vi "Initialise.vi"(8 "error in (no error)":errorcluster, 10 "Message in":refnum<class "InitialiseMessage.lvclass">, 11 "StageSPIM in":refnum<class "StageSPIM.lvclass">) -> (0 "error out":errorcluster, 3 "StageSPIM out":refnum<class "StageSPIM.lvclass">)   [LabVIEW 2012, in "StageSPIM.lvclass"]
doc: "This method is called when an initialise message is received. It mainly initialises the RabbitMQ connectivity. \n\nOverride this method when your component needs special initialisation (e.g. of software or hardware resources). In that case, don't forget to call the parent for proper implementation. If your component owns subcomponents, they count as resources, so you have to initialise them by calling their own initialise functions"
uses:
  StageSPIM.lvclass
  <vilib>/Distrio/Murmex/InitialiseMessage/InitialiseMessage.lvclass
  <vilib>/Distrio/Murmex/Murmex/Murmex.lvclass
  StageSPIM.lvclass/StageSPIM.ctl
panel:
  # "This method is called when the INTIALISE\ntrigger is sent. \n\nOverride this method when your component needs to\nrespond to this trigger. \n\nCall parent for proper implementation"
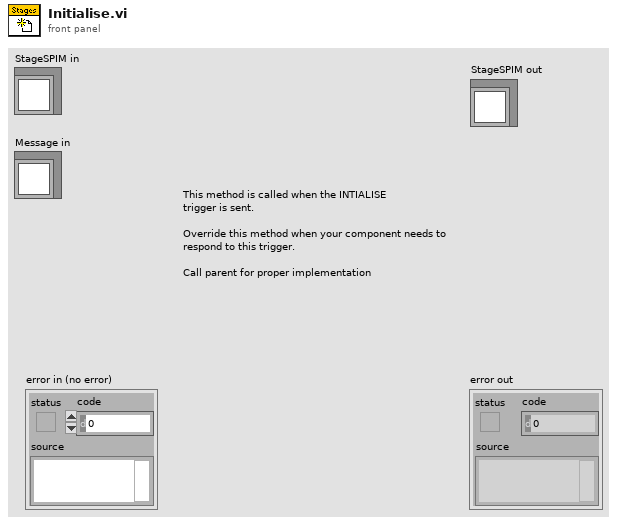
[diagram p1: front panel]
types:
  T1 = cluster{"Register DC":bool, "DaisyChain Search?":bool, "Device ID":i32}[][]
  T2 = cluster{"RON Affected axes":string[], "Reference mode":bool[], "Check FRF?":bool}
  T3 = typedef "StageSPIM.lvclass/port_control.ctl" = i32
  T4 = typedef "StageSPIM.lvclass/baud_rate_control.ctl" = u16
  T5 = typedef "StageSPIM.lvclass/connection_type.ctl" = enum16{"RS232", "RS232 DaisyChain", "USB", "USB_DaisyChain"}
  T6 = cluster{"Register DC":bool, "DaisyChain Search?":bool, "Device ID":i32}
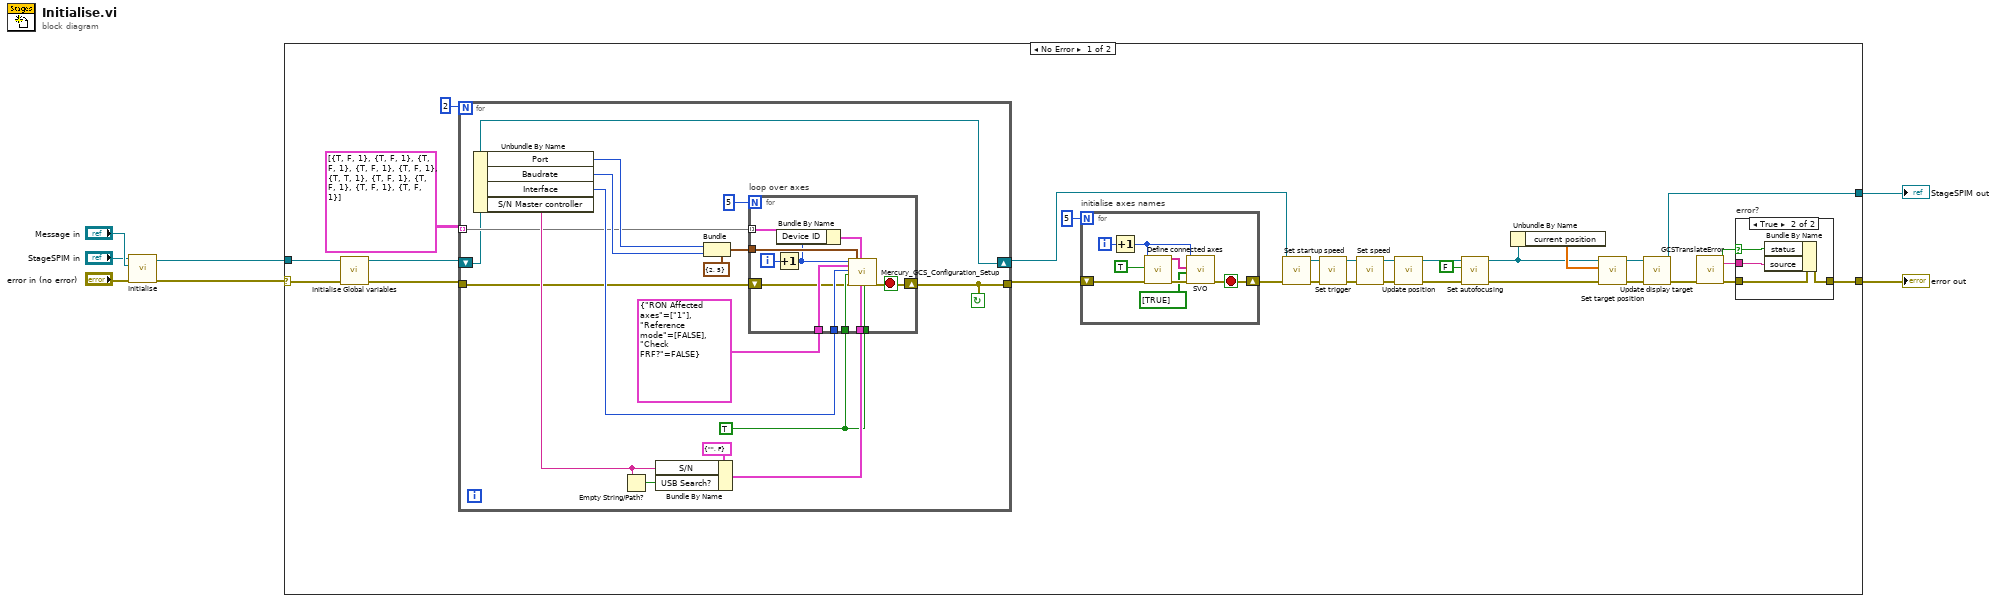
[diagram p0: block diagram]
diagram:
  n1 = call-parent "Initialise.vi"("error in (no error)"="error in (no error)", "Message in"="Message in", "Murmex in"="StageSPIM in") -> ("error out"=w4:errorcluster, "Murmex out"=w3:refnum<class "StageSPIM.lvclass">)  [unwired: 7 in]
  n2 = case shown="No Error" w4 {
    selector: w4 -> [w28 w80]
    tunnel: w3 -> [w26 w79]
    tunnel: [w18 w79] -> w2
    tunnel: [w29 w80] -> w1
    frame No Error {
      n3 = call-dynamic "Initialise Global variables.vi"("error in (no error)"=w28, "StageSPIM in"=w26) -> ("error out"=w27:errorcluster, "StageSPIM out"=w25:refnum<class "StageSPIM.lvclass">)  [unwired: 8 in]
      n4 = for {
        N: 2 -> [_]
        tunnel: [w39] -> w32
        tunnel: w27 -> [w42]
        tunnel: T1 [[{"Register DC"=TRUE, "DaisyChain Search?"=FALSE, "Device ID"=1}, {"Register DC"=TRUE, "DaisyChain Search?"=FALSE, "Device ID"=1}, {"Register DC"=TRUE, "DaisyChain Search?"=FALSE, "Device ID"=1}, {"Register DC"=TRUE, "DaisyChain Search?"=FALSE, "Device ID"=1}, {"Register DC"=TRUE, "DaisyChain Search?"=FALSE, "Device ID"=1}], [{"Register DC"=TRUE, "DaisyChain Search?"=TRUE, "Device ID"=1}, {"Register DC"=TRUE, "DaisyChain Search?"=FALSE, "Device ID"=1}, {"Register DC"=TRUE, "DaisyChain Search?"=FALSE, "Device ID"=1}, {"Register DC"=TRUE, "DaisyChain Search?"=FALSE, "Device ID"=1}, {"Register DC"=TRUE, "DaisyChain Search?"=FALSE, "Device ID"=1}]] -> [w41] mode=indexing
        shift-right: [w40] -> w15
        shift-left: w25 -> [w40]
        stop <- w39 continue-if-true
        w47 = TRUE ("Switch servo on?")
        n5 = Unbundle By Name(w40) -> ("Port"=w45:T3, "Baudrate"=w44:T4, "Interface"=w43:T5, "S/N Master controller"=w49:string)
        n6 = Empty String/Path?(string/path=w49) -> (empty?=w50:bool)
        n7 = Bundle By Name(cluster=cluster{"S/N":string, "USB Search?":bool} {"S/N"="", "USB Search?"=FALSE} ("USB settings"), "S/N"=w49, "USB Search?"=w50) -> (w48:cluster{"S/N":string, "USB Search?":bool})
        n8 = Bundle(cluster=cluster{"Portnumber":i32, "Baudrate":u16} {"Portnumber"=2, "Baudrate"=5} ("RS232 settings"), "Portnumber"=w45, "Baudrate"=w44) -> (w52:cluster{"Portnumber":i32, "Baudrate":u16})
        n9 = for "loop over axes" {
          N: 5 -> [_]
          tunnel: w41 -> [w58] mode=indexing
          tunnel: w43 -> [w65]
          tunnel: w47 -> [w60]
          tunnel: w52 -> [w64]
          tunnel: T2 {"RON Affected axes"=["1"], "Reference mode"=[FALSE], "Check FRF?"=FALSE} ("RON settings") -> [w63]
          tunnel: w48 -> [w62]
          shift-right: [w61] -> w39
          shift-left: w42 -> [w55]
          tunnel: w47 -> [w59]
          i -> [w54]
          stop <- w61 stop-if-true
          n10 = Increment(x=w54) -> (x+1=w56:i32)
          n11 = Bundle By Name(cluster=w58, "Device ID"=w56) -> (w57:T6)
          n12 = call "Mercury_GCS_Configuration_Setup.vi"("System no."=w56, "RON settings"=w63, "Interface"=w65, "All axes?"=w59, "error in"=w55, "RS232 settings"=w64, "DaisyChain settings"=w57, "USB settings"=w62, "Switch servo on?"=w60) -> ("error out"=w61:errorcluster)  [unwired: 4 in, 6 out]
        }
      }
      n13 = for "initialise axes names" {
        N: 5 -> [_]
        shift-right: [w71] -> w17
        shift-left: w32 -> [w78]
        i -> [w76]
        stop <- w71 stop-if-true
        n14 = Increment(x=w76) -> (x+1=w72:i32)
        n15 = call "Define connected axes.vi"("System no."=w72, "Read from\ncontroller?"=TRUE ("Read from\ncontroller?"), "error in"=w78) -> ("Conn. Axes out"=w73:string[], "error out"=w75:errorcluster)  [unwired: 15 in]
        n16 = call "SVO.vi"("System no."=w72, "Axes to command"=w73, "Servo mode"=bool[] [TRUE], "error in"=w75) -> ("error out"=w71:errorcluster)  [unwired: 15 in]
      }
      n17 = call-dynamic "Set startup speed.vi"("error in (no error)"=w17, "StageSPIM in"=w15) -> ("error out"=w16:errorcluster, "StageSPIM out"=w13:refnum<class "StageSPIM.lvclass">)  [unwired: 8 in]
      n18 = call-dynamic "Set trigger.vi"("error in (no error)"=w16, "StageSPIM in"=w13) -> ("error out"=w14:errorcluster, "StageSPIM out"=w12:refnum<class "StageSPIM.lvclass">)  [unwired: 8 in]
      n19 = call-dynamic "Set speed.vi"("error in (no error)"=w14, "StageSPIM in"=w12) -> ("error out"=w30:errorcluster, "StageSPIM out"=w23:refnum<class "StageSPIM.lvclass">)  [unwired: 8 in]
      n20 = call-dynamic "Update position.vi"("error in (no error)"=w30, "StageSPIM in"=w23) -> ("error out"=w24:errorcluster, "StageSPIM out"=w10:refnum<class "StageSPIM.lvclass">)  [unwired: 8 in]
      n21 = call-dynamic "Set autofocusing.vi"("error in (no error)"=w24, "autofocusing?"=FALSE, "StageSPIM in"=w10) -> ("error out"=w11:errorcluster, "StageSPIM out"=w9:refnum<class "StageSPIM.lvclass">)  [unwired: 7 in]
      n22 = Unbundle By Name(w9) -> ("current position"=w20:dbl[])
      n23 = call-dynamic "Set target position.vi"("error in (no error)"=w11, "target position"=w20, "StageSPIM in"=w9) -> ("error out"=w22:errorcluster, "StageSPIM out"=w19:refnum<class "StageSPIM.lvclass">)  [unwired: 7 in]
      n24 = call-dynamic "Update display target.vi"("error in (no error)"=w22, "StageSPIM in"=w19) -> ("error out"=w21:errorcluster, "StageSPIM out"=w18:refnum<class "StageSPIM.lvclass">)  [unwired: 8 in]
      n25 = call "GCSTranslateError.vi"("error in"=w21) -> ("GCS Error?"=w37:bool, "Error Description"=w35:string, "error out"=w36:errorcluster)  [unwired: 16 in]
      n26 = case "error?" shown="True" w37 {
        selector: w37 -> [_ w69]
        tunnel: w36 -> [w66 w70]
        tunnel: w35 -> [_ w68]
        tunnel: [w66 w67] -> w29
        frame False {
        }
        frame True {
          n27 = Bundle By Name(cluster=w70, "status"=w69, "source"=w68) -> (w67:errorcluster)
        }
      }
    }
    frame Error {
    }
  }
  "error out" <- w1
  "StageSPIM out" <- w2
